vi "Start Access Point.vi"(8 "Error In":errorcluster, 11 "EZ430-Chronos Ref":T1) -> (0 "Error Out":errorcluster, 2 "Data":u8[](array[numeric]), 3 "EZ430-Chronos Ref":T1)   [LabVIEW 2011, in "LVH-EZ430.lvlib"]
uses:
  <vilib>/LabVIEW Hacker/LabVIEW Interface for EZ430-Chronos/LVH-EZ430.lvlib
  <vilib>/LabVIEW Hacker/LabVIEW Interface for EZ430-Chronos/Private/Type Defs/EZ430-Chronos Ref.ctl
  <vilib>/LabVIEW Hacker/LabVIEW Interface for EZ430-Chronos/Private/Type Defs/Command.ctl
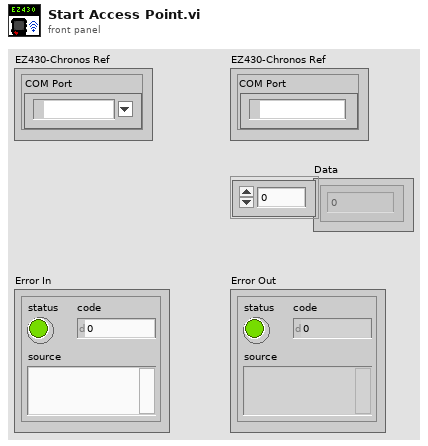
[diagram p1: front panel]
types:
  T1 = typedef "LVH-EZ430.lvlib/EZ430-Chronos Ref.ctl" = cluster{"COM Port":refnum<visa-resource-name>}
  T2 = typedef "LVH-EZ430.lvlib/Command.ctl" = enum8{"Reserved0", "Reserved1", "Reserved2", "Reserved3", "Reserved4", "Reserved5", "Background Polling", "Start Access Point", "Read Accelerometer"}
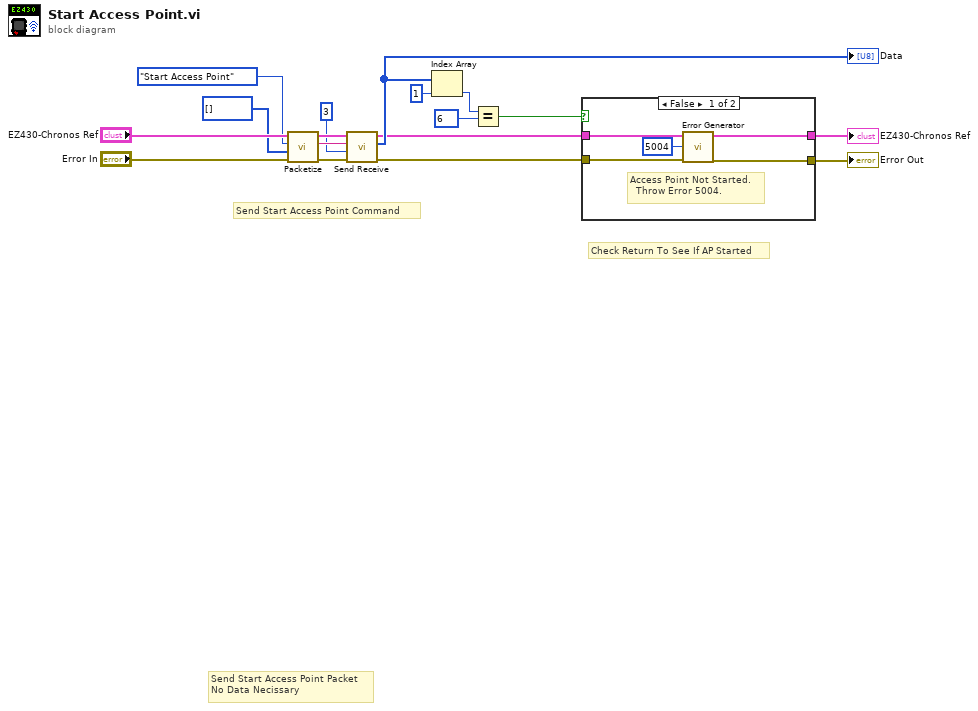
[diagram p0: block diagram]
diagram:
  # "Check Return To See If AP Started"
  # "Send Start Access Point Command"
  # "Send Start Access Point Packet\nNo Data Necissary"
  n1 = call <vilib>:"Packetize.vi"("Error In"="Error In", "Data"=u8[] [], "Command"=Command."Start Access Point", "EZ430-Chronos Config"="EZ430-Chronos Ref") -> ("Error Out"=w14:errorcluster, "Packet"=w12:string, "EZ430-Chronos Config"=w16:T1)  [unwired: 5 in]
  n2 = call <vilib>:"Send Receive.vi"("Error In"=w14, "Bytes To Read"=u32 3, "Packet"=w12, "EZ430-Chronos Config"=w16) -> ("Error Out"=w4:errorcluster, "Data"=w9:u8[], "EZ430-Chronos Config"=w2:T1)  [unwired: 5 in]
  "Data" <- w9
  n3 = Index Array(array=w9, index=1) -> (element=w7:u8)
  n4 = Equal?(x=w7, y=u8 6 ("index")) -> (x = y?=w5:bool)
  n5 = case shown="False" w5 {
    tunnel: w4 -> [w22 w23]
    tunnel: [w21 w23] -> w3
    tunnel: w2 -> [w20 w24]
    tunnel: [w19 w24] -> w1
    frame False {
      # "Access Point Not Started.\n  Throw Error 5004."
      n6 = call <vilib>:"Error Generator.vi"("Error In"=w22, "EZ430-Chronos Error Code"=5004, "EZ430-Chronos Ref"=w20) -> ("Error Out"=w21:errorcluster, "EZ430-Chronos Ref"=w19:T1)  [unwired: 7 in]
    }
    frame True {
      # "Access Point Successfully Started"
    }
  }
  "EZ430-Chronos Ref" <- w1
  "Error Out" <- w3
